vi "GUI.vi"(8 "error in":errorcluster, 11 "Oscilloscope in":refnum<class "Oscilloscope.lvclass">) -> (0 "error out":errorcluster, 3 "Oscilloscope":refnum<class "Oscilloscope.lvclass">)   [LabVIEW 2019, in "Oscilloscope.lvlib" / "Oscilloscope.lvclass"]
uses:
  Oscilloscope.lvclass
  Custom Controls/Horizontal Setting.ctl
  Custom Controls/Trigger Settings.ctl
  Custom Controls/Edge Select.ctl
  Custom Controls/Channel List.ctl
  Custom Controls/Trigger Coupling.ctl
  Custom Controls/Trigger Modifier.ctl
  Custom Controls/Trigger Type.ctl
  Custom Controls/Channel Settings.ctl
  Custom Controls/Vertical Coupling.ctl
  Oscilloscope.lvclass/Oscilloscope.ctl
  Accessors/Read Trigger Settings.vi
  Accessors/Write Active Channel.vi
  Accessors/Read Horizontal Setting.vi
  Accessors/Read Channel Setting.vi
  Accessors/Write Channel Setting.vi
panel:
  in  "Channel List":T1 items=["Channel_1", "Channel_2", "Channel_3", "Channel_4", "Channel_5", "Channel_6", "Channel_7", "Channel_8"]
  in  "Channel Settings":T2={"Amplitude"=0.0, "Vertical Coupling"=enum."DC", "Probe Attenuation"=0.0, "Enable?"=FALSE, "Maximum Input Frequency"=0.0, "Input Impedance"=0, "Timeout (s)"=5.0} {"Timeout (s)" format="%.2f"; "Input Impedance" items=["1 mega ohm", "50 ohms"]; "Maximum Input Frequency" format="%.2f"}
  in  "Trigger":T4={"Edge:"=0, "Level"=0.0, "Source"=0, "trigger coupling"=1, "Holdoff"=0.0, "Delay"=0.0, "Trigger Modifier"=enum."Auto Trigger", "Trigger Type"=enum."Analog Edge"} {"Delay" format="%_6g"; "Holdoff" format="%_6g"; "trigger coupling" items=["AC", "DC", "HF Reject", "LF Reject", "AC Plus HF Reject"]; "Source" items=["Channel_1", "Channel_2", "Channel_3", "Channel_4", "Channel_5", "Channel_6", "Channel_7", "Channel_8"]; "Level" format="%_6g"; "Edge:" items=["Rising Edge", "Falling Edge"]}
  in  "Horizontal Setting":T9={"Num Records"=0, "Sample Rate"=915.5, "Reference Pos"=50.0, "Min Record len"=1000} caption="Horizontal"
  out "Waveform Graph":waveform(dbl)[](graph)
  in  "Active Device":u16(ring)
  in  "stop":bool
  # "Osciloscope"
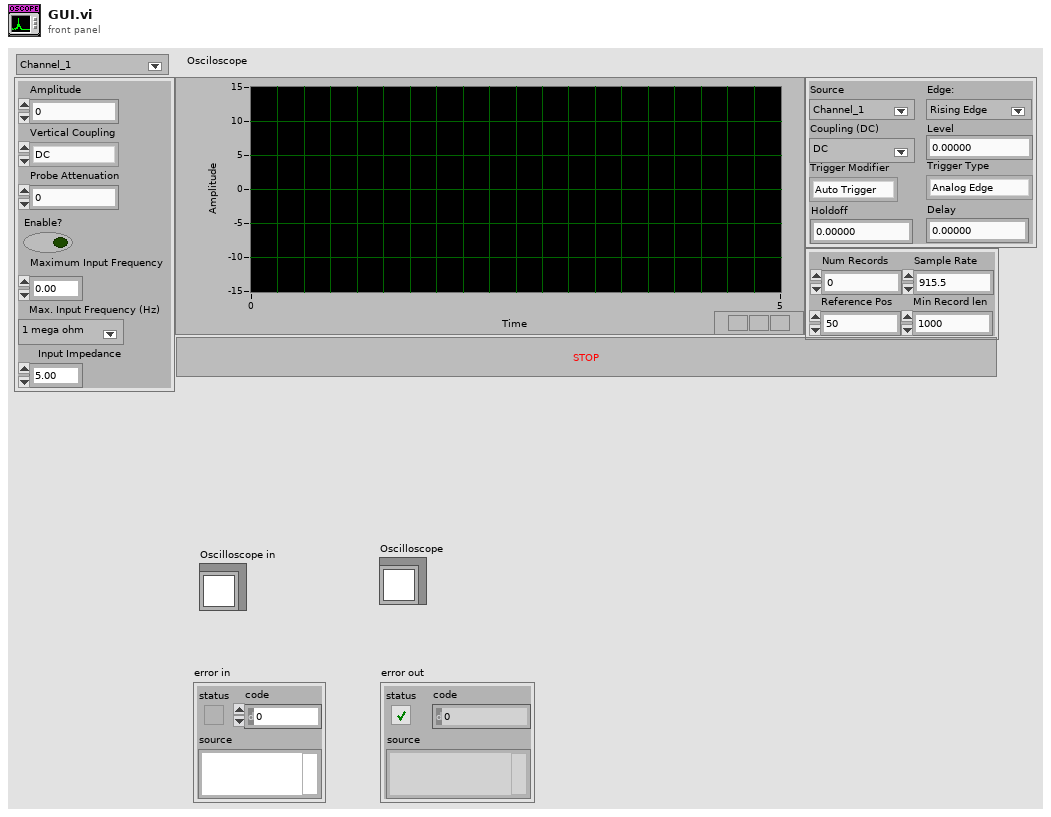
[diagram p1: front panel]
types:
  T1 = typedef "Oscilloscope.lvlib/Oscilloscope.lvclass/Channel List.ctl" = u16
  T2 = typedef "Oscilloscope.lvlib/Oscilloscope.lvclass/Channel Settings.ctl" = cluster{"Amplitude":dbl, "Vertical Coupling":T3, "Probe Attenuation":dbl, "Enable?":bool, "Maximum Input Frequency":dbl, "Input Impedance":u16, "Timeout (s)":dbl}
  T3 = typedef "Oscilloscope.lvlib/Oscilloscope.lvclass/Vertical Coupling.ctl" = enum16{"AC", "DC", "Ground"}
  T4 = typedef "Oscilloscope.lvlib/Oscilloscope.lvclass/Trigger Settings.ctl" = cluster{"Edge:":T5, "Level":dbl, "Source":T1, "trigger coupling":T6, "Holdoff":dbl, "Delay":dbl, "Trigger Modifier":T7, "Trigger Type":T8}
  T5 = typedef "Oscilloscope.lvlib/Oscilloscope.lvclass/Edge Select.ctl" = u16
  T6 = typedef "Oscilloscope.lvlib/Oscilloscope.lvclass/Trigger Coupling.ctl" = u16
  T7 = typedef "Oscilloscope.lvlib/Oscilloscope.lvclass/Trigger Modifier.ctl" = enum16{"Invalid_Setting", "None", "Auto Trigger"}
  T8 = typedef "Oscilloscope.lvlib/Oscilloscope.lvclass/Trigger Type.ctl" = enum16{"Immediate", "Analog Edge", "Digital", "Window", "Hysteresis"}
  T9 = typedef "Oscilloscope.lvlib/Oscilloscope.lvclass/Horizontal Setting.ctl" = cluster{"Num Records":i32, "Sample Rate":dbl, "Reference Pos":dbl, "Min Record len":i32}
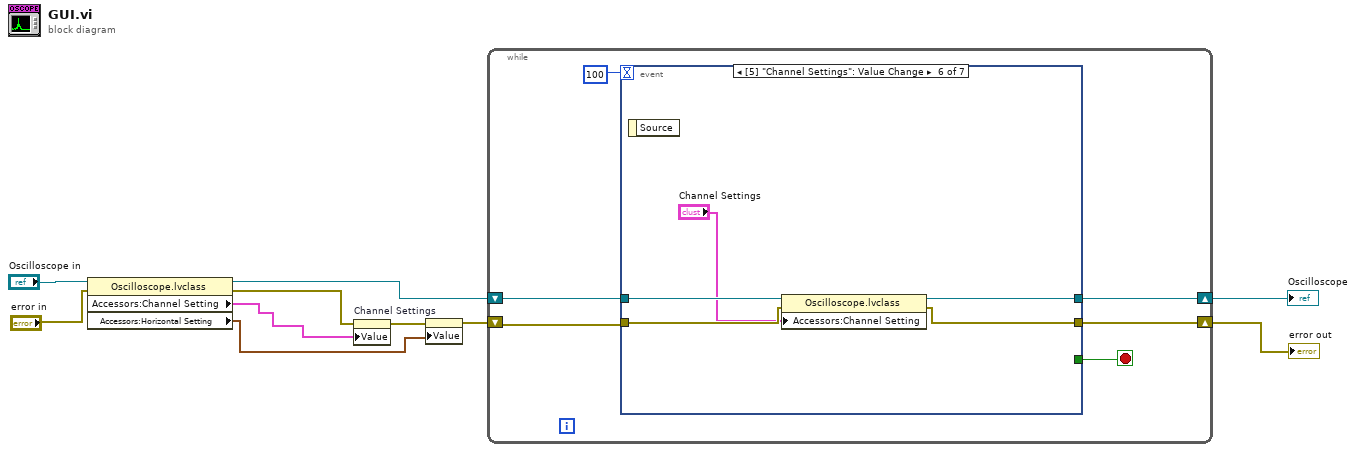
[diagram p0: block diagram]
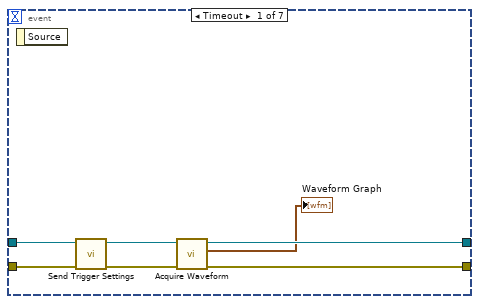
[diagram p2: hidden frame]
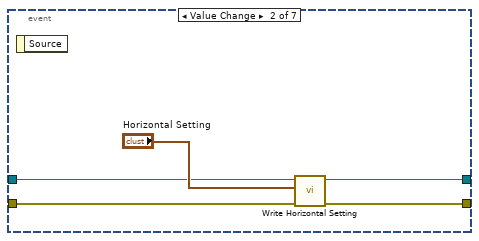
[diagram p3: hidden frame]
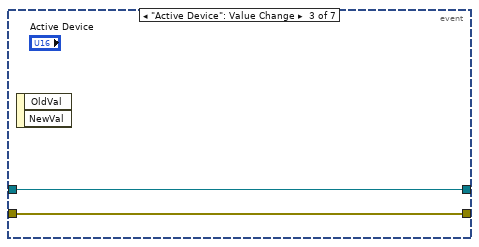
[diagram p4: hidden frame]
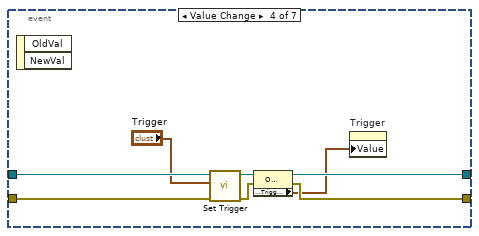
[diagram p5: hidden frame]
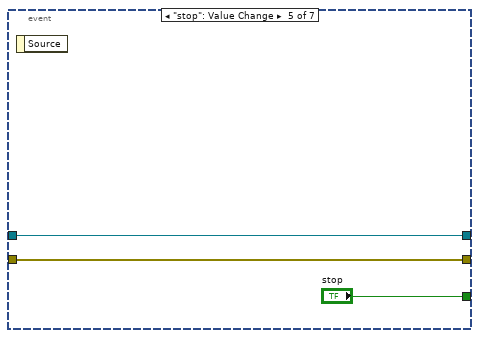
[diagram p6: hidden frame]
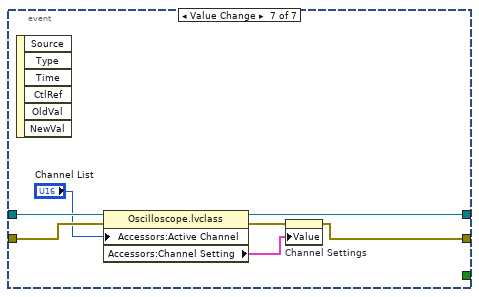
[diagram p7: hidden frame]
diagram:
  n1 = property class="Oscilloscope.lvclass"(reference="Oscilloscope in", error in="error in") -> (reference out=w6:refnum<class "Oscilloscope.lvclass">, error out=w2:errorcluster, "Accessors:Channel Setting"=w1:T2, "Accessors:Horizontal Setting"=w5:T9)
  n2 = property on="Channel Settings" class="Clust (strict)"(error in=w2, "Value"=w1) -> (error out=w3:errorcluster)  [unwired: 1 in, 1 out]
  n3 = property on="Horizontal Setting" class="Clust (strict)"(error in=w3, "Value"=w5) -> (error out=w9:errorcluster)  [unwired: 1 in, 1 out]
  n4 = while {
    shift-right: [w15] -> w4
    shift-left: w6 -> [w16]
    shift-right: [w14] -> w10
    shift-left: w9 -> [w13]
    stop <- w11 stop-if-true
    n5 = event shown="[5] \"Channel Settings\": Value Change" {
      selector: _ -> [_ _ _ _ _ _ _]
      dyn-events: _ -> [_ _ _ _ _ _ _]
      timeout: 100 -> [_ _ _ _ _ _ _]
      tunnel: w16 -> [w19 w25 w30 w37 w41 w46 w53]
      tunnel: [w23 w28 w30 w33 w41 w45 w49] -> w15
      tunnel: [w22 w27 w29 w32 w40 w44 w48] -> w14
      tunnel: w13 -> [w20 w24 w29 w38 w40 w43 w52]
      tunnel: [_ _ _ _ "stop" _ _] -> w11
      event Timeout {
        n6 = event-data() -> ()  [unwired: 1 in, 1 out]
        n7 = call-dynamic "Send Trigger Settings.vi"("error in (no error)"=w20, "Oscilloscope in"=w19) -> ("error out"=w18:errorcluster, "Oscilloscope out"=w17:refnum<class "Oscilloscope.lvclass">)  [unwired: 8 in]
        n8 = call-dynamic "Acquire Waveform.vi"("error in (no error)"=w18, "Oscilloscope in"=w17) -> ("error out"=w22:errorcluster, "Data"=→"Waveform Graph":waveform(dbl)[], "Oscilloscope out"=w23:refnum<class "Oscilloscope.lvclass">)  [unwired: 7 in]
      }
      event Value Change {
        n9 = event-data() -> ()  [unwired: 1 in, 1 out]
        n10 = call "Write Horizontal Setting.vi"("error in (no error)"=w24, "Horizontal Setting"="Horizontal Setting", "Oscilloscope in"=w25) -> ("error out"=w27:errorcluster, "Oscilloscope out"=w28:refnum<class "Oscilloscope.lvclass">)  [unwired: 7 in]
      }
      event "Active Device": Value Change {
        n11 = event-data() -> ()  [unwired: 1 in, 2 out]
      }
      event Value Change {
        n12 = event-data() -> ()  [unwired: 1 in, 2 out]
        n13 = call-dynamic "Set Trigger.vi"("error in (no error)"=w38, "Trigger Settings"="Trigger", "Oscilloscope in"=w37) -> ("error out"=w34:errorcluster, "Oscilloscope out"=w35:refnum<class "Oscilloscope.lvclass">)  [unwired: 7 in]
        n14 = property class="Oscilloscope.lvclass"(reference=w35, error in=w34) -> (reference out=w33:refnum<class "Oscilloscope.lvclass">, error out=w32:errorcluster, "Accessors:Trigger Settings"=w31:T4)
        n15 = property on="Trigger" class="Clust (strict)"("Value"=w31) -> ()  [unwired: 2 in, 2 out]
      }
      event "stop": Value Change {
        n16 = event-data() -> ()  [unwired: 1 in, 1 out]
      }
      event Value Change {
        n17 = event-data() -> ()  [unwired: 1 in, 1 out]
        n18 = property class="Oscilloscope.lvclass"(reference=w46, error in=w43, "Accessors:Channel Setting"="Channel Settings") -> (reference out=w45:refnum<class "Oscilloscope.lvclass">, error out=w44:errorcluster)
      }
      event Value Change {
        n19 = event-data() -> ()  [unwired: 1 in, 6 out]
        n20 = property class="Oscilloscope.lvclass"(reference=w53, error in=w52, "Accessors:Active Channel"="Channel List") -> (reference out=w49:refnum<class "Oscilloscope.lvclass">, error out=w51:errorcluster, "Accessors:Channel Setting"=w50:T2)
        n21 = property on="Channel Settings" class="Clust (strict)"(error in=w51, "Value"=w50) -> (error out=w48:errorcluster)  [unwired: 1 in, 1 out]
      }
    }
  }
  "error out" <- w10
  "Oscilloscope" <- w4
